vi "Filter VIs to Measure.vi"(8 "error in (no error)":errorcluster, 10 "VI Paths":path[](array[path]), 11 "Coverage Analyzer in":refnum<class "Coverage Analyzer.lvclass">) -> (0 "error out":errorcluster, 2 "Filtered VI Paths":path[](array[path]), 3 "Coverage Analyzer out":refnum<class "Coverage Analyzer.lvclass">)   [LabVIEW 2020, in "Coverage Analyzer.lvclass"]
uses:
  Coverage Analyzer.lvclass
  Coverage Analyzer.lvclass/Coverage Analyzer.ctl
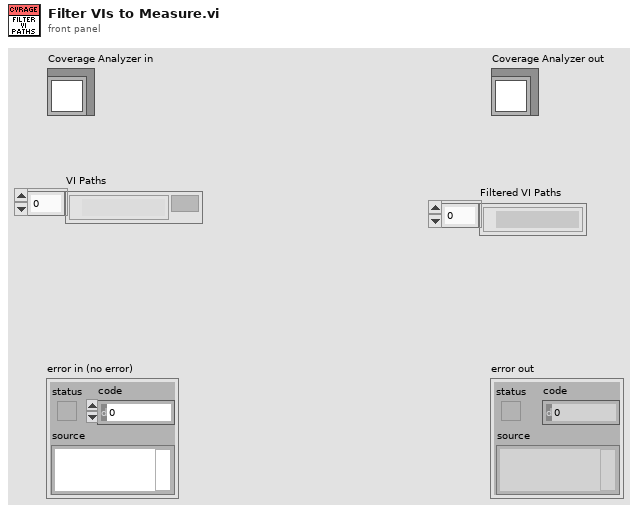
[diagram p1: front panel]
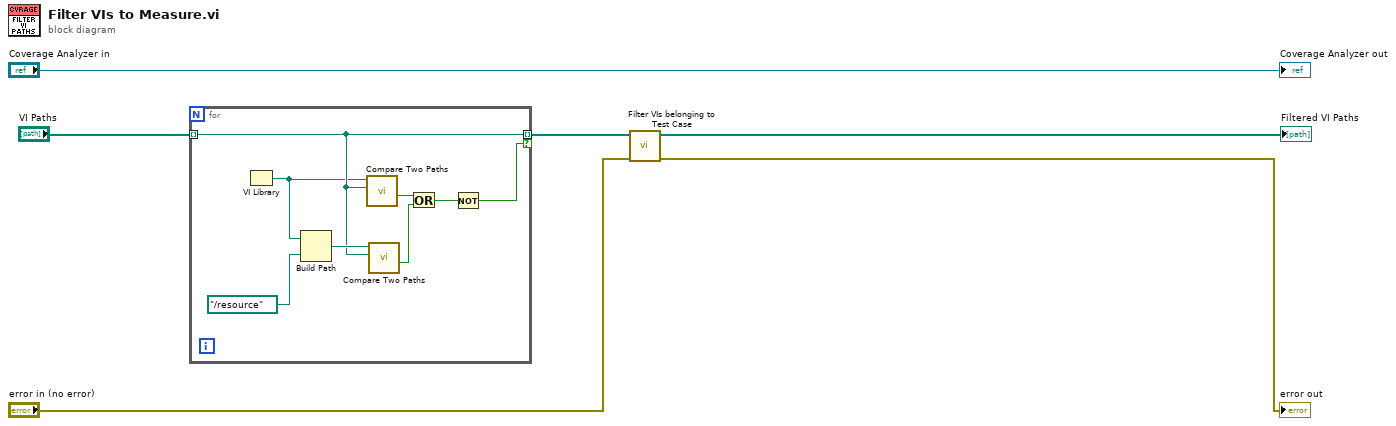
[diagram p0: block diagram]
diagram:
  n1 = for {
    tunnel: "VI Paths" -> [w10] mode=indexing
    tunnel: [w10] -> w4 mode=indexing if=w11
    n2 = VI Library() -> (path=w9:path)
    n3 = Build Path(base path=w9, name or relative path=path "../resource" ("search string")) -> (appended path=w13:path)
    n4 = call <vilib>:"Compare Two Paths.vi"("Path 2"=w10, "Path 1"=w9) -> ("Path 2 Relative to Path 1?"=w12:bool)  [unwired: 6 in, 3 out]
    n5 = call <vilib>:"Compare Two Paths.vi"("Path 2"=w10, "Path 1"=w13) -> ("Path 2 Relative to Path 1?"=w7:bool)  [unwired: 6 in, 3 out]
    n6 = Or(x=w12, y=w7) -> (x .or. y?=w8:bool)
    n7 = Not(x=w8) -> (.not. x?=w11:bool)
  }
  n8 = call "Filter VIs belonging to Test Case.vi"("error in (no error)"="error in (no error)", "Array in"=w4) -> ("error out"=→"error out":errorcluster, "Array out"=→"Filtered VI Paths":path[])  [unwired: 8 in]
  "Coverage Analyzer out" <- "Coverage Analyzer in"
